vi "Handle Command.vi"(8 "error in (no error)":errorcluster, 10 "Data":T1, 11 "DAQmxAI in":refnum<class "DAQmxAI.lvclass">) -> (0 "error out":errorcluster, 3 "DAQmxAI out":refnum<class "DAQmxAI.lvclass">)   [LabVIEW 2023, in "VolatusDAQ.lvlib" / "DAQmxAI.lvclass"]
uses:
  DAQmxAI.lvclass
  DAQmxAI.lvclass/DAQmxAI.ctl
  Volatus/Module/Module.lvclass
  C:/dev/volatus/mts-volatus-super/libs/lv-volatus/Volatus/Module/Module.lvclass
  C:/dev/volatus/mts-volatus-super/libs/lv-volatus/VolatusDAQ/DAQmxAI/DAQmxAI.lvclass
  messages/CmdDigital/Data.ctl
  messages/CmdDigital/CmdDigital.lvlib
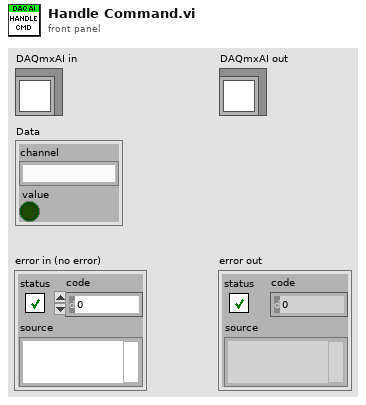
[diagram p1: front panel]
types:
  T1 = typedef "CmdDigital.lvlib/Data.ctl" = cluster{"channel":string, "value":bool}
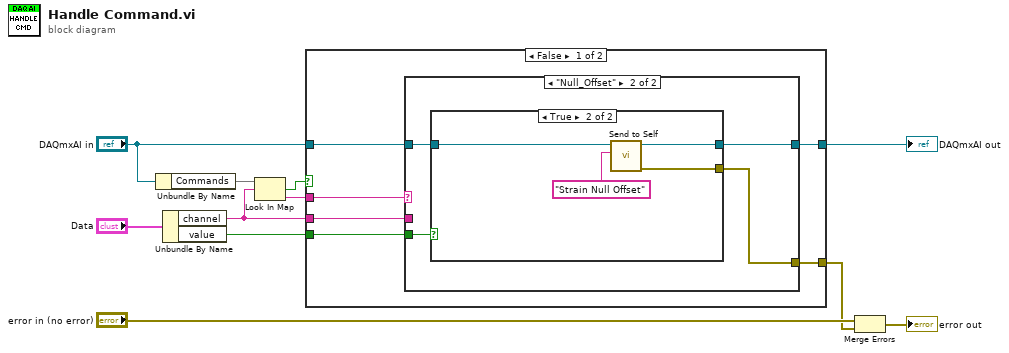
[diagram p0: block diagram]
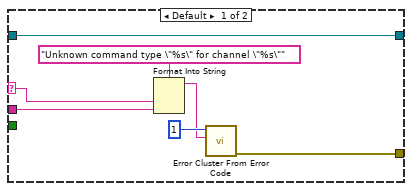
[diagram p2: hidden frame]
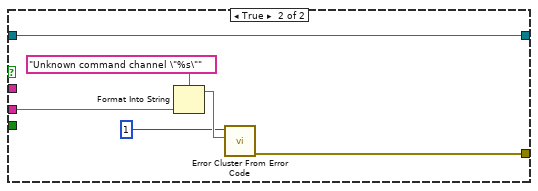
[diagram p4: hidden frame]
diagram:
  n1 = Unbundle By Name("DAQmxAI in") -> ("Commands"=w9:map{string, string})
  n2 = Unbundle By Name("Data") -> ("channel"=w7:string, "value"=w6:bool)
  n3 = Look In Map(map=w9, key=w7) -> (key not found?=w8:bool, value=w5:string)  [unwired: 1 in]
  n4 = case shown="False" w8 {
    tunnel: w7 -> [w16 w39]
    tunnel: w6 -> [w15 _]
    tunnel: [w13 w35] -> w1
    tunnel: w5 -> [w12 _]
    tunnel: "DAQmxAI in" -> [w17 w34]
    tunnel: [w14 w34] -> w3
    frame False {
      n5 = case shown="\"Null_Offset\"" w12 {
        selector: w12 -> [w21 _]
        tunnel: w17 -> [w24 w28]
        tunnel: w16 -> [w22 _]
        tunnel: w15 -> [_ w25]
        tunnel: [w24 w27] -> w14
        tunnel: [w20 w26] -> w13
        frame Default {
          n6 = Format Into String(format string="Unknown command type \"%s\" for channel \"%s\"", w21, w22) -> (resulting string=w18:string)  [unwired: 2 in, 1 out]
          n7 = call <vilib>:"Error Cluster From Error Code.vi"("error message (\"\")"=w18, "error code (0)"=1) -> ("error out"=w20:errorcluster)  [unwired: 7 in]
        }
        frame "Null_Offset" {
          n8 = case shown="True" w25 {
            tunnel: w28 -> [w29 w33]
            tunnel: [w29 w31] -> w27
            tunnel: [_ w30] -> w26
            frame False {
              # "Ignore command to \"un\"trigger."
            }
            frame True {
              n9 = call "Send to Self.vi"("Message ID"="Strain Null Offset", "Module in"=w33) -> ("error out"=w30:errorcluster, "Module out"=w31:refnum<class "DAQmxAI.lvclass">)  [unwired: 8 in]
            }
          }
        }
      }
    }
    frame True {
      n10 = Format Into String(format string="Unknown command channel \"%s\"", w39) -> (resulting string=w37:string)  [unwired: 2 in, 1 out]
      n11 = call <vilib>:"Error Cluster From Error Code.vi"("error message (\"\")"=w37, "error code (0)"=1) -> ("error out"=w35:errorcluster)  [unwired: 7 in]
    }
  }
  "DAQmxAI out" <- w3
  n12 = Merge Errors("error in (no error)", w1) -> (→"error out":errorcluster)
